vi "Cxns-Get Connections File Path.vi"(1 "Connection File Path":path) -> (0 "Path Out":path)   [LabVIEW 2020]
uses:
  <vilib>/Utility/sysdir.llb/System Directory Type.ctl
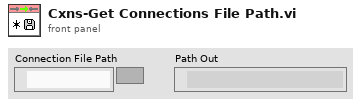
[diagram p1: front panel]
types:
  T1 = typedef "System Directory Type.ctl" = i32
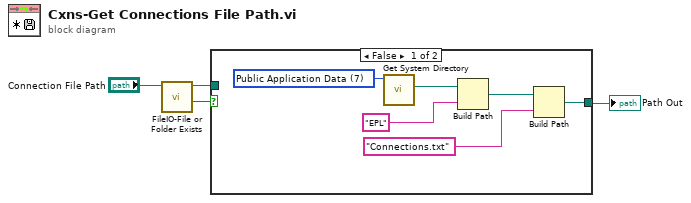
[diagram p0: block diagram]
diagram:
  n1 = call "FileIO-File or Folder Exists.vi"("path"="Connection File Path") -> ("Exists?"=w3:bool, "dup path"=w1:path)  [unwired: 7 in, 2 out]
  n2 = case shown="False" w3 {
    tunnel: w1 -> [_ w11]
    tunnel: [w5 w11] -> w4
    frame False {
      w10 = T1 7 items=["User Home"=0, "User Desktop"=1, "User Documents"=2, "User Application Data"=3, "User Preferences"=4, "User Temporary"=5, "Public Documents"=6, "Public Application Data"=7, "Public Preferences"=8, "Public Cache"=13, "System Core Libraries"=9, "System Installed Libraries"=10, "Application Files"=11, "Boot Volume Root"=12] ("system directory type")
      n3 = call <vilib>:"Get System Directory.vi"("system directory type"=w10) -> ("system directory"=w9:path)  [unwired: 10 in]
      n4 = Build Path(base path=w9, name or relative path="EPL") -> (appended path=w6:path)
      n5 = Build Path(base path=w6, name or relative path="Connections.txt") -> (appended path=w5:path)
    }
    frame True {
    }
  }
  "Path Out" <- w4
